vi "Read Design Log.vi"(6 "Design Log Index":i32, 8 "error in (no error)":errorcluster, 11 "DesignLog":refnum<file>) -> (0 "error out":errorcluster, 1 "Design Inputs":T1={"Q.Plant"=0.0033333333333333335, "C.CoagDoseMax"=0.0, "C.CoagStock"=0.0, "Ti.CoagStock"=0.0, "EN.DrillSeries"=enum."English", "EN.TubeSeries"=enum."English", "N.SedTanks"=0.0, "N.SedBaysEst"=0.0, "W.SedPlate"=0.0, "L.SedPlateSheet"=0.0, "T.SedPlate"=0.0, "T.PlantWall"=0.03, "H.FlocOption"=0.01, "T.FlocBaffleRigidH"=1.7999999999999998, "T.ConcreteMin"=0.3, "T.SedWeir"=0.04, "T.FlocBaffleRigidV"=108000.0} {"T.FlocBaffleRigidV" min=0.0 max=0.2 step=0.001 format="%#.1f"; "T.SedWeir" min=0.001 max=0.2 step=0.001 format="%#.1f"; "T.SedPlate" min=0.001 max=0.05 step=0.001 format="%#.1f"; "T.FlocBaffleRigidH" min=0.0 max=0.2 step=0.001 format="%#.1f"; "T.ConcreteMin" min=0.005 max=0.2 step=0.001 format="%#.1f"; "L.SedPlateSheet" min=0.3 max=8.0 step=0.01 format="%#.1f"; "N.SedBaysEst" min=1.0 max=20.0 step=1.0 format="%#.0f"; "N.SedTanks" min=1.0 max=20.0 step=1.0 format="%#.0f"; "Ti.CoagStock" min=43200.0 max=360000.0 step=3600.0 format="%#.1f"; "H.FlocOption" min=0.5 max=4.0 step=0.01 format="%#.2f"; "C.CoagStock" min=50.0 max=500.0 step=1.0 format="%#.0f"; "C.CoagDoseMax" min=0.03 max=0.2 step=0.005 format="%#.0f"; "Q.Plant" min=0.001 max=0.2 step=0.0001 format="%#.1f"; "T.PlantWall" min=0.05 max=0.5 step=0.001 format="%#.1f"; "W.SedPlate" min=0.5 max=3.0 step=0.001 format="%#.1f"}, 2 "Project inputs":T2, 3 "User Information":T3 {"Country" items=["Afghanistan", "Aland Islands", "Albania", "Algeria", "American Samoa", "Andorra", "Angola", "Anguilla", "Antarctica", "Antigua And Barbuda", "Argentina", "Armenia", "Aruba", "Australia", "Austria", "Azerbaijan", "Bahamas", "Bahrain", "Bangladesh", "Barbados", "Belarus", "Belgium", "Belize", "Benin", "Bermuda", "Bhutan", "Bolivia", "Bosnia And Herzegovina", "Botswana", "Bouvet Island", "Brazil", "British Indian Ocean Territory", "Brunei Darussalam", "Bulgaria", "Burkina Faso", "Burundi", "Cambodia", "Cameroon", "Canada", "Cape Verde", "Cayman Islands", "Central African Republic", "Chad", "Chile", "China", "Christmas Island", "Cocos (Keeling) Islands", "Colombia", "Comoros", "Congo", "Congo, The Democratic Republic Of The", "Cook Islands", "Costa Rica", "Cote D'Ivoire", "Croatia", "Cuba", "Cyprus", "Czech Republic", "Denmark", "Djibouti", "Dominica", "Dominican Republic", "Ecuador", "Egypt", "El Salvador", "Equatorial Guinea", "Eritrea", "Estonia", "Ethiopia", "Falkland Islands (Malvinas)", "Faroe Islands", "Fiji", "Finland", "France", "French Guiana", "French Polynesia", "French Southern Territories", "Gabon", "Gambia", "Georgia", "Germany", "Ghana", "Gibraltar", "Greece", "Greenland", "Grenada", "Guadeloupe", "Guam", "Guatemala", "Guernsey", "Guinea", "Guinea-Bissau", "Guyana", "Haiti", "Heard Island And Mcdonald Islands", "Holy See (Vatican City State)", "Honduras", "Hong Kong", "Hungary", "Iceland", "India", "Indonesia", "Iran, Islamic Republic Of", "Iraq", "Ireland", "Isle Of Man", "Israel", "Italy", "Jamaica", "Japan", "Jersey", "Jordan", "Kazakhstan", "Kenya", "Kiribati", "Korea, Democratic People'S Republic Of", "Korea, Republic Of", "Kuwait", "Kyrgyzstan", "Lao People'S Democratic Republic", "Latvia", "Lebanon", "Lesotho", "Liberia", "Libyan Arab Jamahiriya", "Liechtenstein", "Lithuania", "Luxembourg", "Macao", "Macedonia, The Former Yugoslav Republic Of", "Madagascar", "Malawi", "Malaysia", "Maldives", "Mali", "Malta", "Marshall Islands", "Martinique", "Mauritania", "Mauritius", "Mayotte", "Mexico", "Micronesia, Federated States Of", "Moldova, Republic Of", "Monaco", "Mongolia", "Montserrat", "Morocco", "Mozambique", "Myanmar", "Namibia", "Nauru", "Nepal", "Netherlands", "Netherlands Antilles", "New Caledonia", "New Zealand", "Nicaragua", "Niger", "Nigeria", "Niue", "Norfolk Island", "Northern Mariana Islands", "Norway", "Oman", "Pakistan", "Palau", "Palestinian Territory, Occupied", "Panama", "Papua New Guinea", "Paraguay", "Peru", "Philippines", "Pitcairn", "Poland", "Portugal", "Puerto Rico", "Qatar", "Reunion", "Romania", "Russian Federation", "Rwanda", "Saint Helena", "Saint Kitts And Nevis", "Saint Lucia", "Saint Pierre And Miquelon", "Saint Vincent And The Grenadines", "Samoa", "San Marino", "Sao Tome And Principe", "Saudi Arabia", "Senegal", "Serbia And Montenegro", "Seychelles", "Sierra Leone", "Singapore", "Slovakia", "Slovenia", "Solomon Islands", "Somalia", "South Africa", "South Georgia And The South Sandwich Islands", "Spain", "Sri Lanka", "Sudan", "Suriname", "Svalbard And Jan Mayen", "Swaziland", "Sweden", "Switzerland", "Syrian Arab Republic", "Taiwan, Province Of China", "Tajikistan", "Tanzania, United Republic Of", "Thailand", "Timor-Leste", "Togo", "Tokelau", "Tonga", "Trinidad And Tobago", "Tunisia", "Turkey", "Turkmenistan", "Turks And Caicos Islands", "Tuvalu", "Uganda", "Ukraine", "United Arab Emirates", "United Kingdom", "United States", "United States Minor Outlying Islands", "Uruguay", "Uzbekistan", "Vanuatu", "Venezuela", "Viet Nam", "Virgin Islands, British", "Virgin Islands, U.S.", "Wallis And Futuna", "Western Sahara", "Yemen", "Zambia", "Zimbabwe", "(Not Specified)"]}, 4 "Last Design":i32, 5 "Date":string)   [LabVIEW 2015]
uses:
  User Information.ctl
  Country Ring.ctl
  Project inputs.ctl
  Basic Inputs.ctl
  AguaClara Library.lvlib
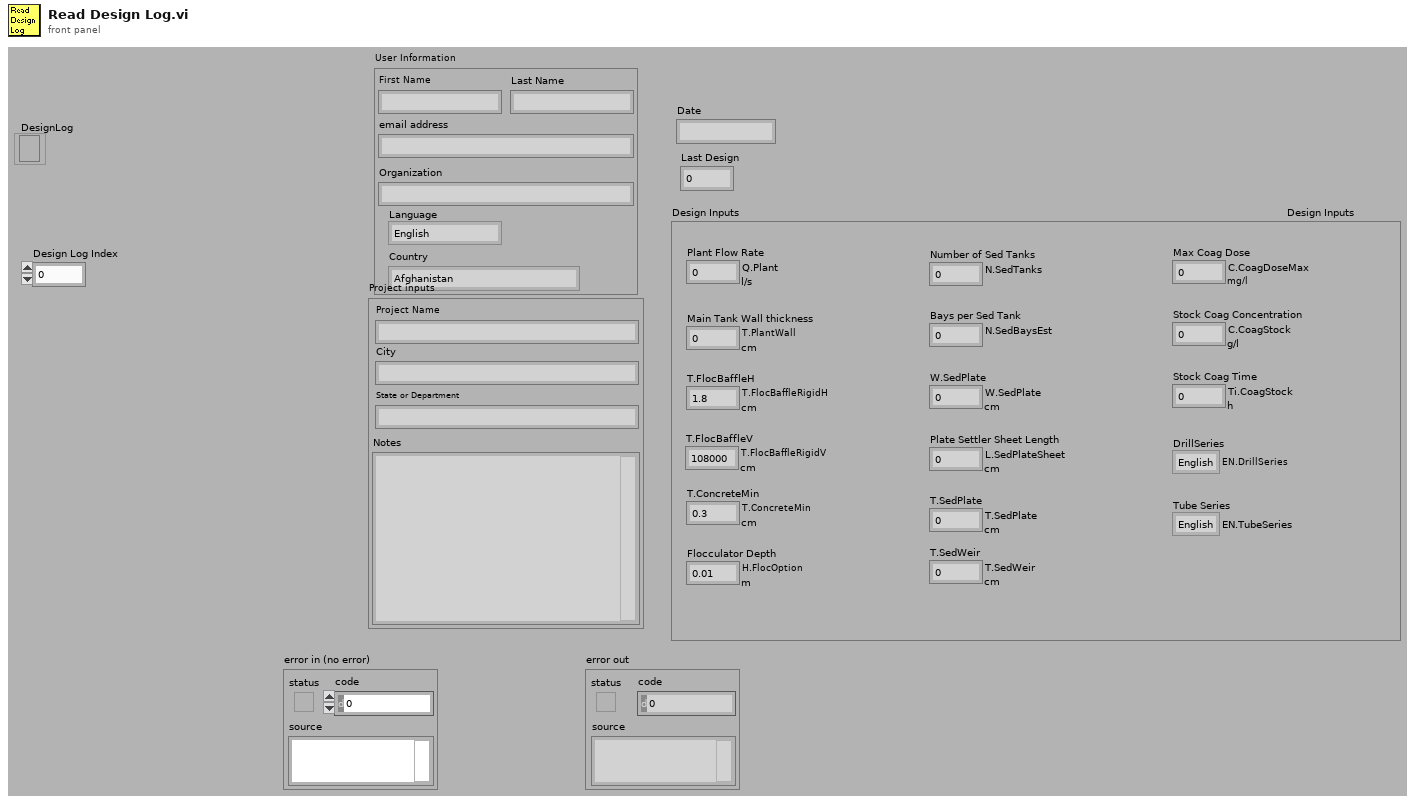
[diagram p1: front panel]
types:
  T1 = typedef "AguaClara Library.lvlib/Basic Inputs.ctl" = cluster{"Q.Plant":dbl[unit], "C.CoagDoseMax":dbl[unit], "C.CoagStock":dbl[unit], "Ti.CoagStock":dbl[unit], "EN.DrillSeries":enum16{"English", "Metric"}, "EN.TubeSeries":enum16{"English", "Metric"}, "N.SedTanks":dbl, "N.SedBaysEst":dbl, "W.SedPlate":dbl[unit], "L.SedPlateSheet":dbl[unit], "T.SedPlate":dbl[unit], "T.PlantWall":dbl[unit], "H.FlocOption":dbl[unit], "T.FlocBaffleRigidH":dbl[unit], "T.ConcreteMin":dbl[unit], "T.SedWeir":dbl[unit], "T.FlocBaffleRigidV":dbl[unit]}
  T2 = typedef "AguaClara Library.lvlib/Project inputs.ctl" = cluster{"Project Name":string, "City":string, "State":string, "Notes":string}
  T3 = typedef "AguaClara Library.lvlib/User Information.ctl" = cluster{"First Name":string, "Last Name":string, "Email Address":string, "Organization":string, "Language":enum16{"English", "Español", "French"}, "Country":T4}
  T4 = typedef "Country Ring.ctl" = u16
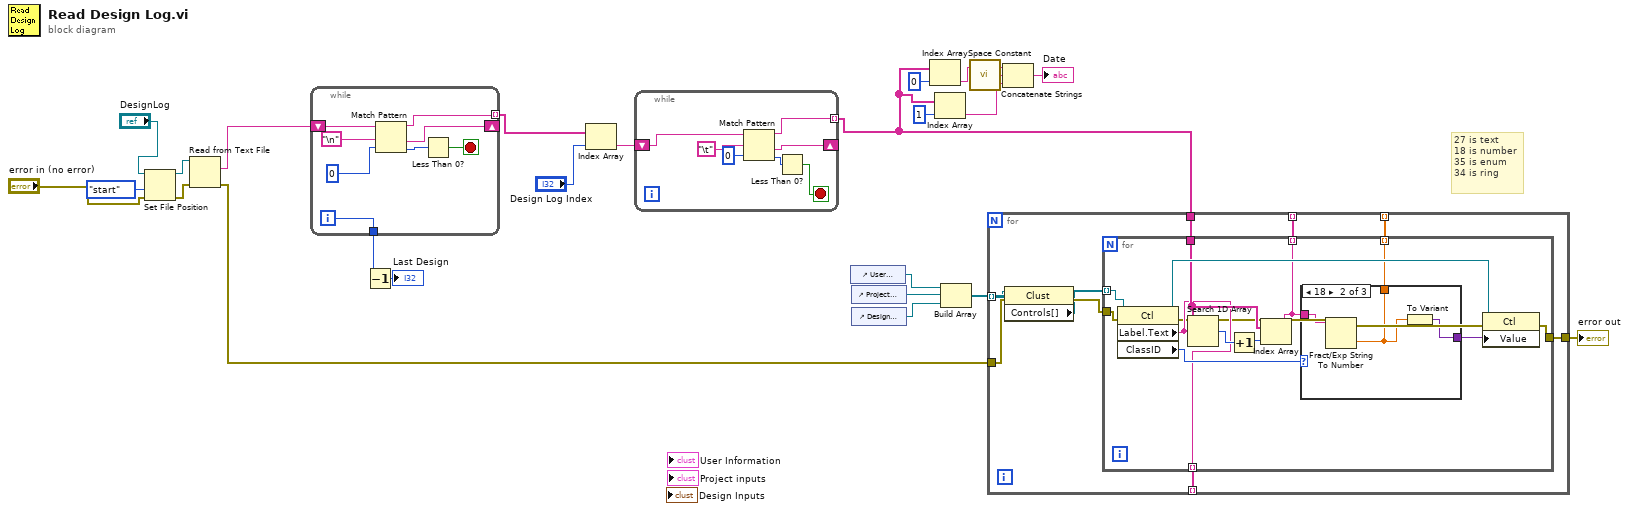
[diagram p0: block diagram]
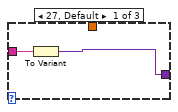
[diagram p2: hidden frame]
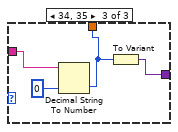
[diagram p3: hidden frame]
diagram:
  # "27 is text\n18 is number\n35 is enum\n34 is ring"
  n1 = Set File Position(refnum="DesignLog", from (0:start)=enum16{"start", "end", "current"}."start", error in="error in (no error)") -> (refnum out=w2:refnum<file>, error out=w6:errorcluster)  [unwired: 1 in]
  n2 = Read from Text File(file (use dialog)=w2, error in=w6) -> (text=w24:string, error out=w4:errorcluster)  [unwired: 2 in, 2 out]
  n3 = while {
    shift-right: [w31] -> _
    shift-left: w24 -> [w32]
    tunnel: [w30] -> w23 mode=indexing
    tunnel: [w25] -> w8
    i -> [w25]
    stop <- w27 stop-if-true
    n4 = Match Pattern(string=w32, regular expression="\n", offset (0)=0 ("offset past match")) -> (before substring=w30:string, after substring=w31:string, offset past match=w28:i32)  [unwired: 1 out]
    n5 = Less Than 0?(x=w28) -> (x < 0?=w27:bool)
  }
  n6 = Decrement(x=w8) -> (x-1=→"Last Design":i32)
  n7 = Index Array(array=w23, index="Design Log Index") -> (element=w21:string)
  n8 = while {
    shift-right: [w33] -> _
    shift-left: w21 -> [w39]
    tunnel: [w34] -> w13 mode=indexing
    stop <- w35 stop-if-true
    n9 = Match Pattern(string=w39, regular expression="\t", offset (0)=0) -> (before substring=w34:string, after substring=w33:string, offset past match=w36:i32)  [unwired: 1 out]
    n10 = Less Than 0?(x=w36) -> (x < 0?=w35:bool)
  }
  n11 = control-ref of="User Information"() -> (w20:refnum<vi>)
  n12 = control-ref of="Project inputs"() -> (w18:refnum<vi>)
  n13 = control-ref of="Design Inputs"() -> (w17:refnum<vi>)
  n14 = Index Array(array=w13, index=0) -> (element=w12:string)
  n15 = Index Array(array=w13, index=1) -> (element=w11:string)
  n16 = Build Array(w20, w18, w17) -> (w19:refnum<vi>[])
  n17 = call <vilib>:"Space Constant.vi"() -> ("String"=w10:string)
  n18 = for {
    tunnel: w19 -> [w48] mode=indexing
    tunnel: w13 -> [w45]
    tunnel: [w44] -> _ mode=indexing
    tunnel: [w43] -> _ mode=indexing
    tunnel: [w42] -> _ mode=indexing
    tunnel: w4 -> [w41]
    tunnel: [w40] -> w16
    n19 = property class="Clust"(reference=w48, error in=w41) -> (error out=w47:errorcluster, "Controls[]"=w46:refnum<vi>[])  [unwired: 1 out]
    n20 = for {
      tunnel: w47 -> [w61]
      tunnel: w46 -> [w60] mode=indexing
      tunnel: w45 -> [w56]
      tunnel: [w53] -> w44 mode=indexing
      tunnel: [w52] -> w43 mode=indexing
      tunnel: [w51] -> w42 mode=indexing
      tunnel: [w49] -> w40
      n21 = property class="Ctl"(reference=w60, error in=w61) -> (reference out=w59:refnum<vi>, error out=w50:errorcluster, "Label.Text"=w52:string, "ClassID"=w55:u32)
      n22 = Search 1D Array(1D array=w56, element=w52) -> (index of element=w58:i32)  [unwired: 1 in]
      n23 = Increment(x=w58) -> (x+1=w57:i32)
      n24 = Index Array(array=w56, index=w57) -> (element=w53:string)
      n25 = case shown="18" w55 {
        tunnel: w53 -> [w63 w65 w70]
        tunnel: [w62 w66 w68] -> w54
        tunnel: [_ w64 w67] -> w51
        frame 27, Default {
          n26 = To Variant(anything=w63) -> (Variant=w62:variant)
        }
        frame 18 {
          n27 = Fract/Exp String To Number(string=w65) -> (number=w64:dbl)  [unwired: 3 in, 1 out]
          n28 = To Variant(anything=w64) -> (Variant=w66:variant)
        }
        frame 34, 35 {
          n29 = Decimal String To Number(string=w70, default (0L)=0) -> (number=w67:i32)  [unwired: 1 in, 1 out]
          n30 = To Variant(anything=w67) -> (Variant=w68:variant)
        }
      }
      n31 = property class="Ctl"(reference=w59, error in=w50, "Value"=w54) -> (error out=w49:errorcluster)  [unwired: 1 out]
    }
  }
  "error out" <- w16
  n32 = Concatenate Strings(w12, w10, w11) -> (→"Date":string)
